vi "CheesyDrive.vi"(6 "Quickturn":bool, 9 "Sensitivty":dbl=1.0, 10 "Wheel":dbl(slide) scale=-1.0..1.0, 11 "Throttle":dbl(slide)=0.007874015748031496 scale=-1.0..1.0) -> (2 "Right PWM":dbl, 3 "Left PWM":dbl)   [LabVIEW 2016]
panel:
  in  "Max dx/dt":dbl=7.0
  in  "QuickStop?":bool=TRUE
  in  "alpha":dbl=0.1
  out "Waveform Chart":dbl(graph)
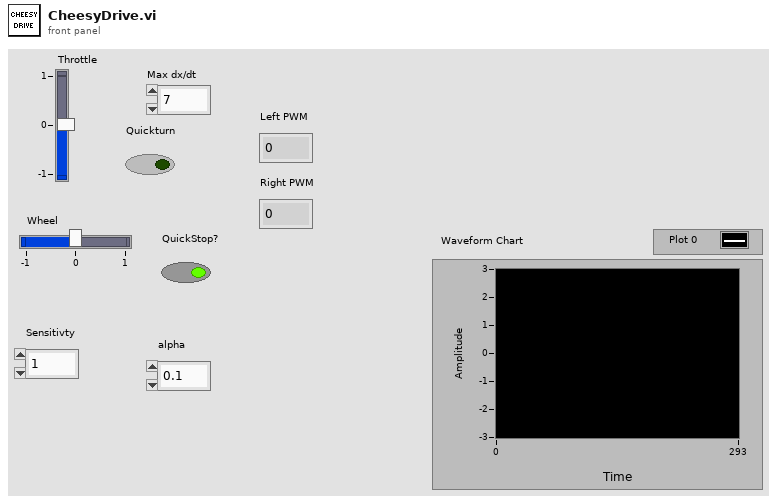
[diagram p1: front panel]
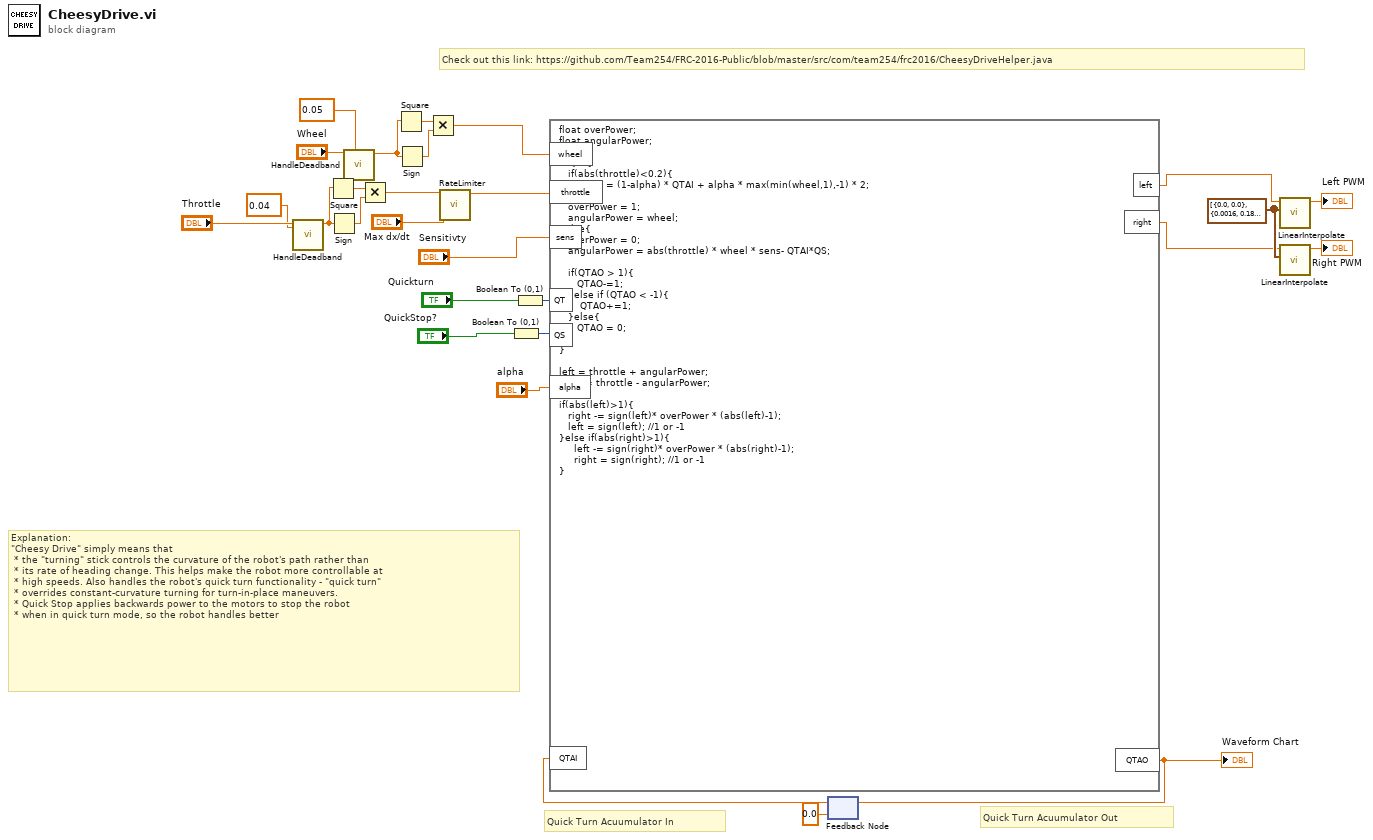
[diagram p0: block diagram]
diagram:
  w14 = cluster{"X":dbl, "Y":dbl}[] [{"X"=0.0, "Y"=0.0}, {"X"=0.0016, "Y"=0.185}, {"X"=1.0, "Y"=1.0}] ("Points")
  # "Explanation:\n\"Cheesy Drive\" simply means that\n * the \"turning\" stick controls the curvature of the robot's path rather than\n * its rate of heading change. This helps make the robot more controllable at\n * high speeds. Also handles the robot's quick turn functionality - \"quick turn\"\n * overrides constant-curvature turning for turn-in-place maneuvers.\n * Quick Stop applies backwards power to the motors to stop the robot\n * when in quick turn mode, so the robot handles better"
  # "Quick Turn Acuumulator Out"
  # "Quick Turn Acuumulator In"
  # "Check out this link: https://github.com/Team254/FRC-2016-Public/blob/master/src/com/team254/frc2016/CheesyDriveHelper.java"
  n1 = call "HandleDeadband.vi"("Deadband"=0.04, "Input"="Throttle") -> ("Output"=w16:dbl)  [unwired: 9 in]
  n2 = Square(x=w16) -> (x^2=w17:dbl)
  n3 = Sign(1:w16) -> (0:w15:dbl)
  n4 = call "HandleDeadband.vi"("Deadband"=0.05, "Input"="Wheel") -> ("Output"=w2:dbl)  [unwired: 9 in]
  n5 = Multiply(x=w17, y=w15) -> (x*y=w7:dbl)
  n6 = Square(x=w2) -> (x^2=w3:dbl)
  n7 = Sign(1:w2) -> (0:w4:dbl)
  n8 = Multiply(x=w3, y=w4) -> (x*y=w1:dbl)
  n9 = call "RateLimiter.vi"("Max dx/dt"="Max dx/dt", "Input"=w7) -> ("Output"=w6:dbl)  [unwired: 9 in]
  n10 = Boolean To (0,1)(Boolean="QuickStop?") -> (0, 1=w8:i16)
  n11 = Boolean To (0,1)(Boolean="Quickturn") -> (0, 1=w21:i16)
  n12 = feedback #1(0.0 ("QTAccumulatorO")) -> (w19:dbl)
  n13 = formula code="float overPower;\nfloat angularPower;\n\nif(QT){\n   if(abs(throttle)<0.2){\n      QTAO = (1-alpha) * QTAI + alpha * max(min(wheel,1),-1) * 2;\n   }\n   overPower = 1;\n   angularPower = wheel;\n}else{\n   overPower = 0;\n   angularPower = abs(throttle) * wheel * sens- QTAI*QS;\n\n   if(QTAO > 1){\n      QTAO-=1;\n   }else if (QTAO < -1){\n       QTAO+=1;\n   }else{\n      QTAO = 0;\n  }\n}\n\nleft = throttle + angularPower;\nright = throttle - angularPower;\n\nif(abs(left)>1){\n   right -= sign(left)* overPower * (abs(left)-1);\n   left = sign(left); //1 or -1\n}else if(abs(right)>1){\n     left -= sign(right)* overPower * (abs(right)-1);\n     right = sign(right); //1 or -1 \n}"("wheel"=w1, "throttle"=w6, "sens"="Sensitivty", "QT"=w21, "alpha"="alpha", "QTAI"=w19, "QS"=w8) -> ("left"=w12:dbl, "right"=w13:dbl, "QTAO"=w22:dbl)
  "Waveform Chart" <- w22
  n14 = feedback-in #1(w22) -> ()
  n15 = call "LinearInterpolate.vi"("Points"=w14, "Value"=w12) -> ("Output"=→"Left PWM":dbl)  [unwired: 9 in]
  n16 = call "LinearInterpolate.vi"("Points"=w14, "Value"=w13) -> ("Output"=→"Right PWM":dbl)  [unwired: 9 in]
